vi "LJLogM read and log.vi"(0 "Data File Reference In":path, 1 "# Channels":i32=4 min=1 max=16, 2 "Row Modification Options":T1={" Row #"=1, "Delete Row"=FALSE, "Insert Row"=FALSE} {"Row #" min=0 max=95}, 3 "Max File Size (Bytes)":i32=1048576 min=1 max=2000000000, 4 "Channel Setup Reference In":refnum<vi>, 5 "Error In":errorcluster, 6 "Handle In":i32, 7 "Update Channel Ref":bool, 8 "Data File Prefix":string="data", 9 "Write to file Selected?":bool, 10 "Working Directory":path, 12 "Is Log Interval?":bool) -> (11 "Error Message Status":bool, 13 "Error Message":string="No Error", 14 "Data File Reference Out":path=path "None", 15 "Handle Out":i32, 16 "Raw Data":dbl[](array[numeric]), 17 "Scaled Data":dbl[](array[numeric]), 18 "Channel Setup Reference Out":refnum<vi>, 19 "(LJM) Error Out":errorcluster)   [LabVIEW 2026]
uses:
  Common Logger Controls/Channel Setup.ctl
  Common Logger Controls/Row Modification Options.ctl
panel:
  in  "Channel Setup":T2={"Name"=["AIN0", "AIN1", "AIN2", "AIN3", "AIN4", "AIN5", "AIN6", "AIN7", "AIN8", "AIN9", "AIN10", "AIN11", "AIN12", "AIN13", "AIN14", "AIN15", "AIN16", "AIN17", "AIN18", "AIN19", "AIN20", "AIN21", "AIN22", "AIN23", "AIN24", "AIN25", "AIN26", "AIN27", "AIN28", "AIN29", "AIN30", "AIN31", "AIN32", "AIN33", "AIN34", "AIN35", "AIN36", "AIN37", "AIN38", "AIN39", "AIN40", "AIN41", "AIN42", "AIN43", "AIN44", "AIN45", "AIN46", "AIN47", "AIN48", "AIN49", "AIN50", "AIN51", "AIN52", "AIN53", "AIN54", "AIN55", "AIN56", "AIN57", "AIN58", "AIN59", "AIN60", "AIN61", "AIN62", "AIN63", "AIN64", "AIN65", "AIN66", "AIN67", "AIN68", "AIN69", "AIN70", "AIN71", "AIN72", "AIN73", "AIN74", "AIN75", "AIN76", "AIN77", "AIN78", "AIN79", "AIN80", "AIN81", "AIN82", "AIN83", "AIN84", "AIN85", "AIN86", "AIN87", "AIN88", "AIN89", "AIN90", "AIN91", "AIN92", "AIN93", "AIN94", "AIN95", "AIN96", "AIN97", "AIN98", "AIN99"], "", "Scaling Equation"=["y=a", "y=b", "y=c", "y=d", "y=e", "y=f", "y=g", "y=h", "y=i", "y=j", "y=k", "y=l", "y=m", "y=n", "y=o", "y=p", "y=a2", "y=b2", "y=c2", "y=d2", "y=e2", "y=f2", "y=g2", "y=h2", "y=i2", "y=j2", "y=k2", "y=l2", "y=m2", "y=n2", "y=o2", "y=p2", "y=a3", "y=b3", "y=c3", "y=d3", "y=e3", "y=f3", "y=g3", "y=h3", "y=i3", "y=j3", "y=k3", "y=l3", "y=m3", "y=n3", "y=o3", "y=p3", "y=a4", "y=b4", "y=c4", "y=d4", "y=e4", "y=f4", "y=g4", "y=h4", "y=i4", "y=j4", "y=k4", "y=l4", "y=m4", "y=n4", "y=o4", "y=p4", "y=a5", "y=b5", "y=c5", "y=d5", "y=e5", "y=f5", "y=g5", "y=h5", "y=i5", "y=j5", "y=k5", "y=l5", "y=m5", "y=n5", "y=o5", "y=p5", "y=a6", "y=b6", "y=c6", "y=d6", "y=e6", "y=f6", "y=g6", "y=h6", "y=i6", "y=j6", "y=k6", "y=l6", "y=m6", "y=n6", "y=o6", "y=p6", "y=a7", "y=b7", "y=c7", "y=d7"], "", "Graph?"=[TRUE, TRUE, TRUE, TRUE, FALSE, FALSE, FALSE, FALSE, FALSE, FALSE, FALSE, FALSE, FALSE, FALSE, FALSE, FALSE, FALSE, FALSE, FALSE, FALSE, FALSE, FALSE, FALSE, FALSE, FALSE, FALSE, FALSE, FALSE, FALSE, FALSE, FALSE, FALSE, FALSE, FALSE, FALSE, FALSE, FALSE, FALSE, FALSE, FALSE, FALSE, FALSE, FALSE, FALSE, FALSE, FALSE, FALSE, FALSE, FALSE, FALSE, FALSE, FALSE, FALSE, FALSE, FALSE, FALSE, FALSE, FALSE, FALSE, FALSE, FALSE, FALSE, FALSE, FALSE, FALSE, FALSE, FALSE, FALSE, FALSE, FALSE, FALSE, FALSE, FALSE, FALSE, FALSE, FALSE, FALSE, FALSE, FALSE, FALSE, FALSE, FALSE, FALSE, FALSE, FALSE, FALSE, FALSE, FALSE, FALSE, FALSE, FALSE, FALSE, FALSE, FALSE, FALSE, FALSE, FALSE, FALSE, FALSE, FALSE]}
  # "0"
  # "1"
  # "2"
  # "3"
  # "4"
  # "5"
  # "6"
  # "7"
  # "8"
  # "9"
  # "10"
  # "11"
  # "12"
  # "13"
  # "14"
  # "15"
  # "16"
  # "17"
  # "18"
  # "19"
  # "20"
  # "21"
  # "22"
  # "23"
  # "24"
  # "25"
  # "26"
  # "27"
  # "28"
  # "29"
  # "30"
  # "31"
  # "32"
  # "33"
  # "34"
  # "35"
  # "36"
  # "37"
  # "38"
  # "39"
  # "40"
  # "41"
  # "42"
  # "43"
  # "44"
  # "45"
  # "46"
  # "47"
  # "48"
  # "49"
  # "50"
  # "51"
  # "52"
  # "53"
  # "54"
  # "55"
  # "56"
  # "57"
  # "58"
  # "59"
  # "60"
  # "61"
  # "62"
  # "63"
  # "64"
  # "65"
  # "66"
  # "67"
  # "68"
  # "69"
  # "70"
  # "71"
  # "72"
  # "73"
  # "74"
  # "75"
  # "76"
  # "77"
  # "78"
  # "79"
  # "80"
  # "81"
  # "82"
  # "83"
  # "84"
  # "85"
  # "86"
  # "87"
  # "88"
  # "89"
  # "90"
  # "91"
  # "92"
  # "93"
  # "94"
  # "95"
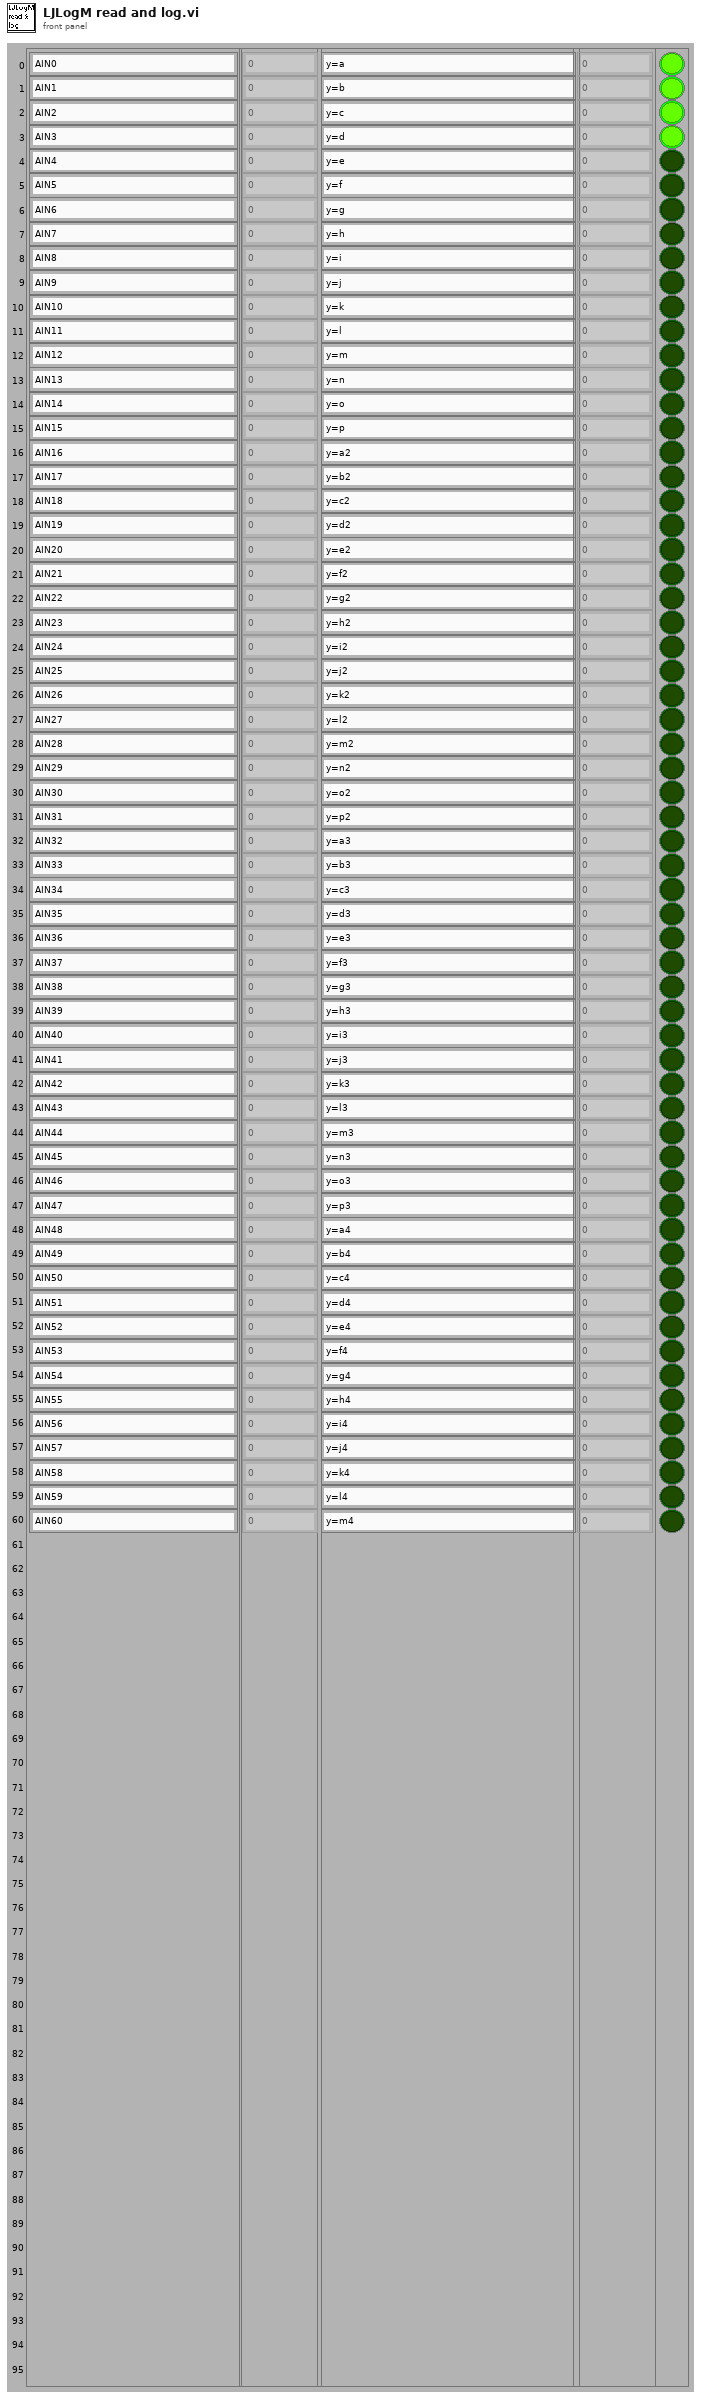
[diagram p1: front panel]
types:
  T1 = typedef "Row Modification Options.ctl" = cluster{" Row #":i32, "Delete Row":bool, "Insert Row":bool}
  T2 = typedef "Channel Setup.ctl" = cluster{"Name":string[], string, "Scaling Equation":string[], string, "Graph?":bool[]}
  T3 = cluster{"Name":string[], string, "Scaling Equation":string[], string, "Graph?":bool[]}
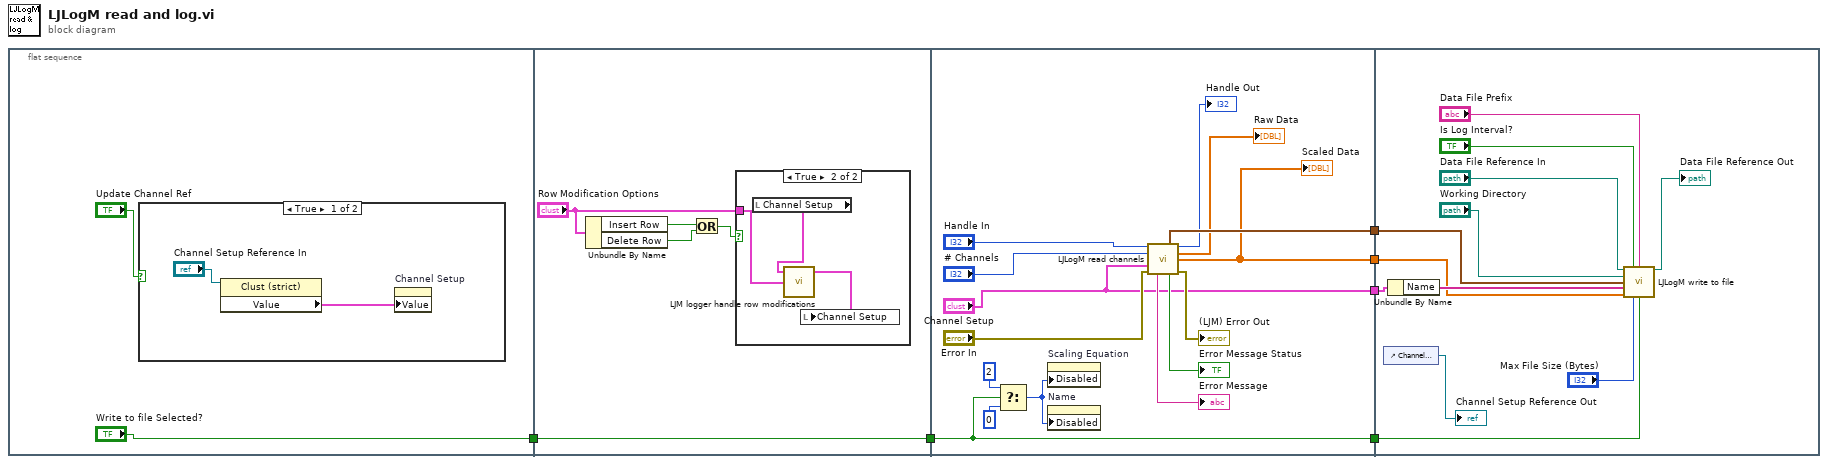
[diagram p0: block diagram]
diagram:
  n1 = flat-sequence {
    tunnel: ["Write to file Selected?"] -> w2
    tunnel: w2 -> [w15]
    tunnel: [w15] -> w1
    tunnel: [w33] -> w6
    tunnel: [w32] -> w5
    tunnel: ["Channel Setup"] -> w4
    tunnel: [w21] -> w3
    tunnel: w1 -> [w21]
    tunnel: w6 -> [w36]
    tunnel: w5 -> [w39]
    tunnel: w4 -> [w38]
    tunnel: w3 -> [w35]
    frame #0 {
      n2 = case shown="True" "Update Channel Ref" {
        frame True {
          n3 = property class="Clust (strict)"(reference="Channel Setup Reference In") -> ("Value"=w9:T3)  [unwired: 1 in, 2 out]
          n4 = property on="Channel Setup" class="Clust (strict)"("Value"=w9) -> ()  [unwired: 2 in, 2 out]
        }
        frame False {
        }
      }
    }
    frame #1 {
      n5 = Unbundle By Name("Row Modification Options") -> ("Insert Row"=w11:bool, "Delete Row"=w12:bool)
      n6 = Or(x=w11, y=w12) -> (x .or. y?=w13:bool)
      n7 = case shown="True" w13 {
        tunnel: "Row Modification Options" -> [_ w18]
        frame False {
        }
        frame True {
          n8 = local read "Channel Setup"() -> (w16:T2)
          n9 = call "LJM logger handle row modifications.vi"("Row Modification Options"=w18, "Channel Setup"=w16) -> ("Channel Setup Out"=w17:T2)  [unwired: 3 in]
          n10 = local write "Channel Setup"(w17) -> ()
        }
      }
    }
    frame #2 {
      n11 = Select(t=u8 2 ("Disabled"), s=w21, f=u8 0 ("Disabled")) -> (s? t:f=w20:u8)
      n12 = property on="Scaling Equation" class="Arr (strict)"("Disabled"=w20) -> ()  [unwired: 2 in, 2 out]
      n13 = property on="Name" class="Arr (strict)"("Disabled"=w20) -> ()  [unwired: 2 in, 2 out]
      n14 = call "LJLogM read channels.vi"("Handle In"="Handle In", "# Channels"="# Channels", "Channel Setup In"="Channel Setup", "Error In"="Error In") -> ("Timestamp"=w33:timestamp, "Handle Out"=→"Handle Out":i32, "Raw Data"=→"Raw Data":dbl[], "Scaled Data"=w32:dbl[], "Error Message"=→"Error Message":string, "Error Message Status"=→"Error Message Status":bool, "(LJM) Error Out"=→"(LJM) Error Out":errorcluster)  [unwired: 5 in]
      "Scaled Data" <- w32
    }
    frame #3 {
      n15 = control-ref of="Channel Setup"() -> (→"Channel Setup Reference Out":refnum<vi>)
      n16 = Unbundle By Name(w38) -> ("Name"=w43:string[])
      n17 = call "LJLogM write to file.vi"("Data File Reference In"="Data File Reference In", "Is Log Interval?"="Is Log Interval?", "Data File Prefix"="Data File Prefix", "Working Directory"="Working Directory", "Timestamp"=w36, "Channel Names"=w43, "Channel Data"=w39, "Max File Size (Bytes)"="Max File Size (Bytes)", "Write to file?"=w35) -> ("Data File Reference Out"=→"Data File Reference Out":path)  [unwired: 5 in, 1 out]
    }
  }
